vi "Treshold_Finder_V2.vi"(3 "IMM":u16[](array[numeric]), 4 "IPR's":dbl) -> (0 "OMM":u16[](array[numeric]), 1 "DAC Value":i32, 2 "Condicion":bool)   [LabVIEW 2012]
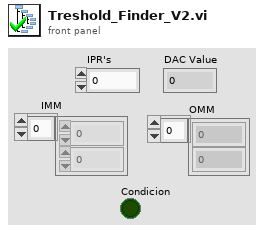
[diagram p1: front panel]
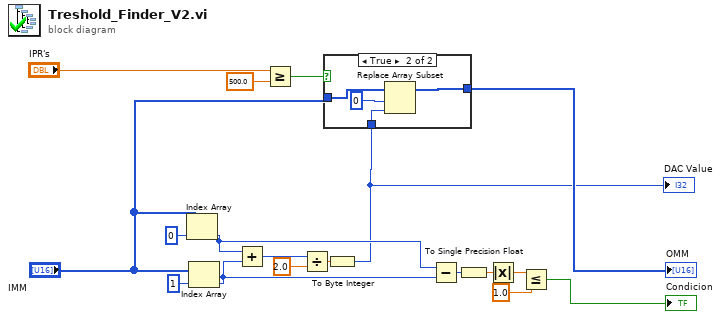
[diagram p0: block diagram]
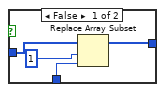
[diagram p2: hidden frame]
diagram:
  n1 = Index Array(array="IMM", index=0) -> (element=w9:u16)
  n2 = Index Array(array="IMM", index=1) -> (element=w8:u16)
  n3 = Add(x=w9, y=w8) -> (x+y=w14:u16)
  n4 = Greater Or Equal?(x="IPR's", y=500.0) -> (x >= y?=w11:bool)
  n5 = Divide(x=w14, y=2.0) -> (x/y=w10:dbl)
  n6 = To Byte Integer(number=w10) -> (8bit integer=w2:i8)
  "DAC Value" <- w2
  n7 = case shown="True" w11 {
    tunnel: "IMM" -> [w20 w25]
    tunnel: [w19 w26] -> w18
    tunnel: w2 -> [w22 w23]
    frame False {
      n8 = Replace Array Subset(array=w20, new element=w22, index=1) -> (w19:u16[])
    }
    frame True {
      n9 = Replace Array Subset(array=w25, new element=w23, index=0) -> (w26:u16[])
    }
  }
  "OMM" <- w18
  n10 = Subtract(x=w9, y=w8) -> (x-y=w7:u16)
  n11 = To Single Precision Float(number=w7) -> (single precision float=w6:sgl)
  n12 = Absolute Value(x=w6) -> (abs(x)=w5:sgl)
  n13 = Less Or Equal?(x=w5, y=sgl 1.0) -> (x <= y?=→"Condicion":bool)
